vi "Set Top Level VI.vi"(8 "error in (no error)":errorcluster, 11 "teststand-api in":refnum<class "teststand-api.lvclass">) -> (0 "error out":errorcluster, 3 "teststand-api out":refnum<class "teststand-api.lvclass">)   [LabVIEW 2014, in "teststand-api.lvlib" / "teststand-api.lvclass"]
uses:
  teststand-api.lvclass
  teststand-api.lvclass/teststand-api.ctl
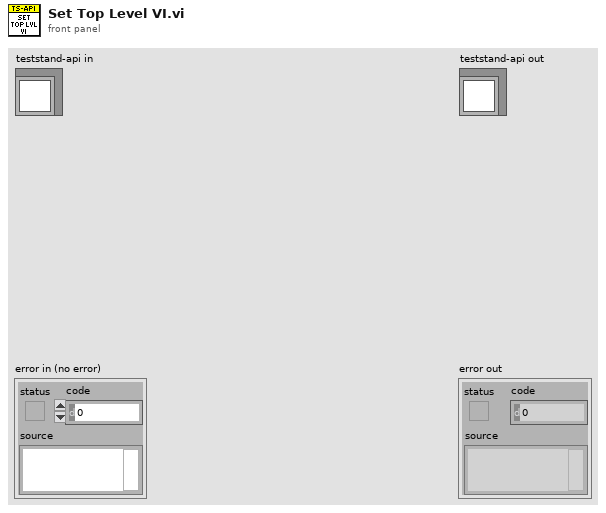
[diagram p1: front panel]
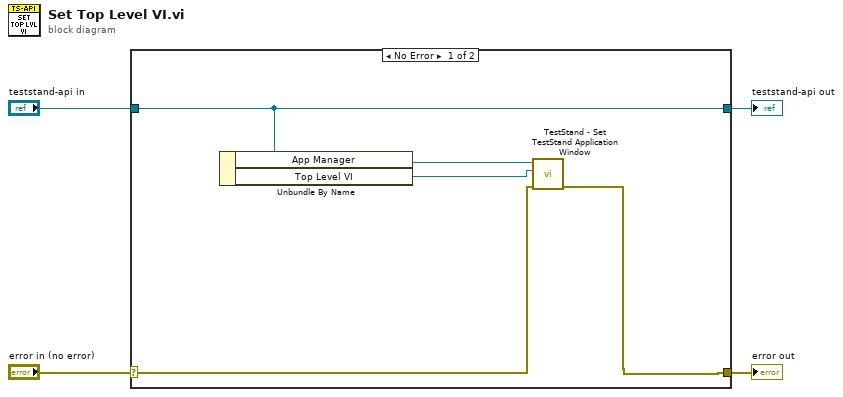
[diagram p0: block diagram]
diagram:
  n1 = case shown="No Error" "error in (no error)" {
    selector: "error in (no error)" -> [w7 w11]
    tunnel: [w6 w11] -> w3
    tunnel: [w9 w10] -> w1
    tunnel: "teststand-api in" -> [w9 w10]
    frame No Error {
      n2 = Unbundle By Name(w9) -> ("App Manager"=w8:refnum<k7>, "Top Level VI"=w5:refnum<vi>)
      n3 = call <vilib>:"TestStand - Set TestStand Application Window.vi"("error in (no error)"=w7, "VI Refnum (Caller's Refnum)"=w5, "Application Manager"=w8) -> ("error out"=w6:errorcluster)  [unwired: 8 in]
    }
    frame Error {
    }
  }
  "error out" <- w3
  "teststand-api out" <- w1
